vi "Core Destroy.vi"(8 "error in (no error)":errorcluster, 11 "CIFTemplateNode in":refnum<class "CIFCorePlugin.lvclass">) -> (0 "error out":errorcluster, 3 "CIFTemplateNode out":refnum<class "CIFCorePlugin.lvclass">)   [LabVIEW 2021, in "CIFCorePlugin.lvclass"]
uses:
  CIFCorePlugin.lvclass
  CIFCorePlugin.lvclass/CIFCorePlugin.ctl
  CIFCoreOOB/OOB_Rx/CIFCoreOOB_Rx.lvclass
  D:/dev/CIF-LVCore/src/CIFUtilities/CIFOutOfBand/CIFOutOfBand.lvclass
  CIFCoreOOB/OOB_Tx/CIFCoreOOB_Tx.lvclass
  CIFCoreGrpc/CIFCorePlugin_server/RPC Service/PluginCore/PluginCore.lvclass
  CIFUtilities/CIFClocks/Core/Get Time.vi
  CIFCoreCommon/Utilities/Update Delta Time.vi
  Accessors/Timestamps/Read Destroying TS.vi
  Accessors/Get Time.vi
  CIFUtilities/CIFClocks/Time Conversion/LabVIEW Time to UTC Time.vi
  CIFUtilities/CIFClocks/SubVIs/Add Error.vi
  CIFCoreCommon/Utilities/Append Error Location.vi
  Logs/Log State Change.vi
  CIFUtilities/CIFOutOfBand/CIFOutOfBand.lvclass
  D:/dev/CIF-LVCore/src/CIFCore/CIFCoreOOB/OOB_Rx/CIFCoreOOB_Rx.lvclass
  D:/dev/CIF-LVCore/src/CIFCore/CIFCoreOOB/OOB_Tx/CIFCoreOOB_Tx.lvclass
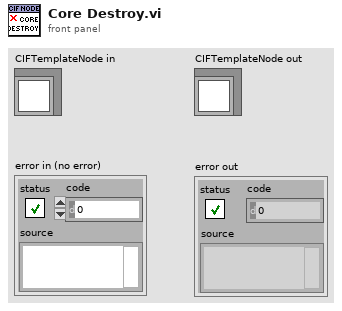
[diagram p1: front panel]
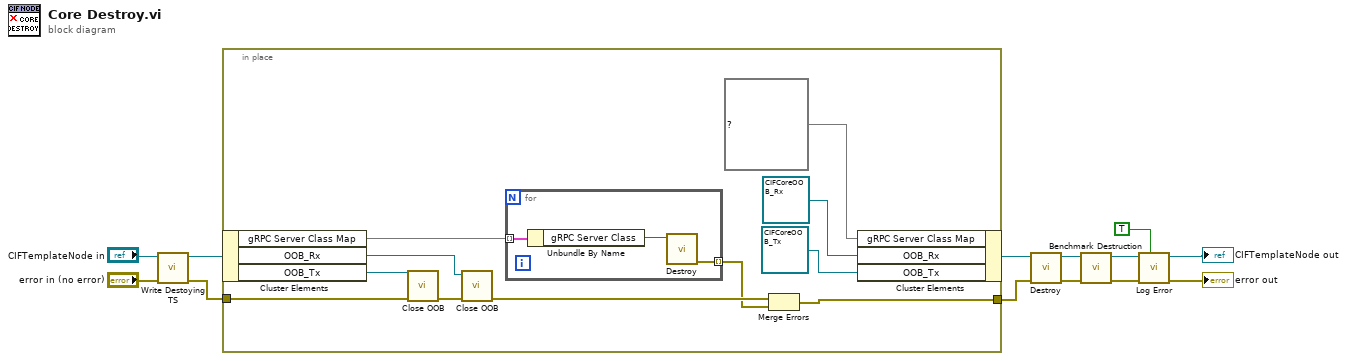
[diagram p0: block diagram]
diagram:
  n1 = call "Write Destoying TS.vi"("error in (no error)"="error in (no error)", "CIFCorePlugin in"="CIFTemplateNode in") -> ("error out"=w7:errorcluster, "CIFCorePlugin out"=w8:refnum<class "CIFCorePlugin.lvclass">)  [unwired: 8 in]
  n2 = in-place {
    in-place-border: w7 -> [w24]
    in-place-border: [w17] -> w12
    n3 = in-place-cluster #1(w8) -> ("gRPC Server Class Map"=w20:map{string, refnum<class "PluginCore.lvclass">}, "OOB_Rx"=w22:refnum<class "CIFCoreOOB_Rx.lvclass">, "OOB_Tx"=w21:refnum<class "CIFCoreOOB_Tx.lvclass">)
    n4 = call "Close OOB.vi"("error in"=w24, "OOB in"=w21) -> ("error out"=w23:errorcluster)  [unwired: 9 in]
    n5 = call "Close OOB.vi"("error in"=w23, "OOB in"=w22) -> ("error out"=w19:errorcluster)  [unwired: 9 in]
    n6 = for {
      tunnel: w20 -> [w27] mode=indexing
      tunnel: [w25] -> w18 mode=indexing
      n7 = Unbundle By Name(w27) -> ("gRPC Server Class"=w26:refnum<class "PluginCore.lvclass">)
      n8 = call-dynamic "Destroy.vi"("SignalGeneratorService in"=w26) -> ("error out"=w25:errorcluster)  [unwired: 9 in, 1 out]
    }
    n9 = Merge Errors(w19, w18) -> (w17:errorcluster)
    n10 = in-place-cluster #1("gRPC Server Class Map"=map{string, refnum<class "PluginCore.lvclass">} {}, "OOB_Rx"=refnum<class "CIFCoreOOB_Rx.lvclass"> refnum, "OOB_Tx"=refnum<class "CIFCoreOOB_Tx.lvclass"> refnum) -> (w13:refnum<class "CIFCorePlugin.lvclass">)
  }
  n11 = call-dynamic "Destroy.vi"("error in (no error)"=w12, "CIFTemplateNode in"=w13) -> ("error out"=w10:errorcluster, "CIFTemplateNode out"=w11:refnum<class "CIFCorePlugin.lvclass">)  [unwired: 8 in]
  n12 = call "Benchmark Destruction.vi"("error in (no error)"=w10, "CIFCorePlugin in"=w11) -> ("error out"=w4:errorcluster, "CIFCorePlugin out"=w5:refnum<class "CIFCorePlugin.lvclass">)  [unwired: 8 in]
  n13 = call "Log Error.vi"("Write to Terminal"=TRUE, "error in (no error)"=w4, "CIFCorePlugin in"=w5) -> ("error out"=→"error out":errorcluster, "CIFCorePlugin out"=→"CIFTemplateNode out":refnum<class "CIFCorePlugin.lvclass">)  [unwired: 7 in]
